vi "ParsePerformance.vi"(0 "data out":string, 1 "offset":u8) -> (2 "pckTotal":u32, 3 "pckSuccess":u32, 4 "timestamp":u32)   [LabVIEW 2009]
panel:
  out "Bytes Read":i32
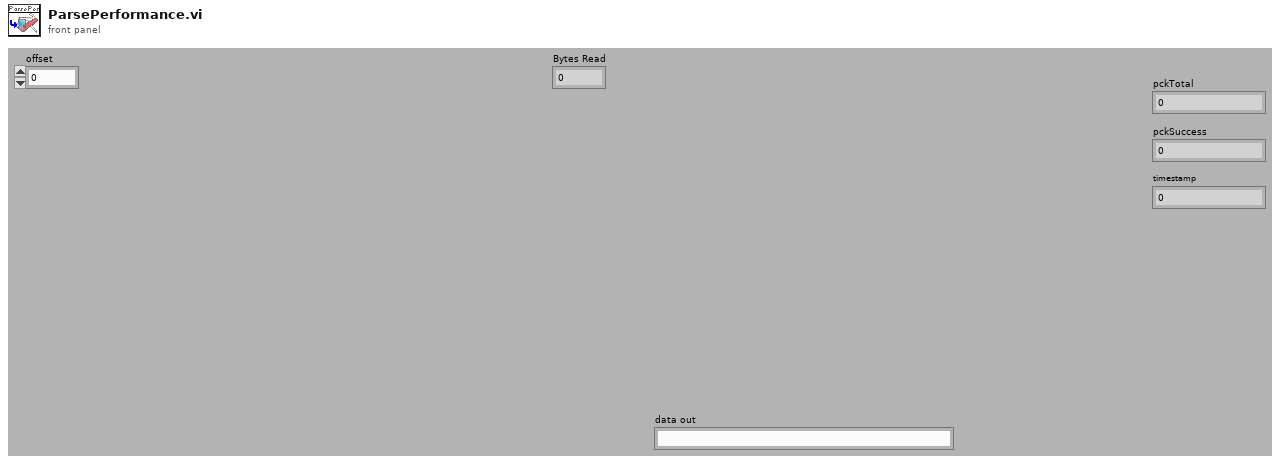
[diagram p1: front panel]
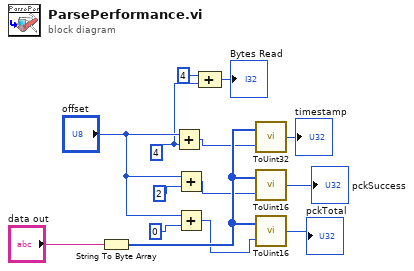
[diagram p0: block diagram]
diagram:
  w3 = 4 ("index")
  n1 = String To Byte Array(string="data out") -> (unsigned byte array=w13:u8[])
  n2 = Add(x="offset", y=w3) -> (x+y=w4:i32)
  n3 = Add(x="offset", y=2 ("index")) -> (x+y=w5:i32)
  n4 = Add(x="offset", y=0 ("index")) -> (x+y=w6:i32)
  n5 = Compound Arithmetic op=unknown(4 ("value"), w3) -> (→"Bytes Read":i32)
  n6 = call "ToUint32.vi"("index"=w4, "array"=w13) -> ("sp float"=→"timestamp":u32)
  n7 = call "ToUint16.vi"("index"=w5, "array"=w13) -> ("sp float"=→"pckSuccess":u16)
  n8 = call "ToUint16.vi"("index"=w6, "array"=w13) -> ("sp float"=→"pckTotal":u16)
